vi "getparam.vi"(8 "error in (no error)":errorcluster, 11 "Input":string="34,45,89") -> (0 "error out":errorcluster, 3 "Output":string)   [LabVIEW 2014]
uses:
  <userlib>/Nanonis Prog Interface V5/Scan/Piezos/Piezo Calibration Range Get.vi
  <userlib>/Nanonis Prog Interface V5/Nanonis Prog Interface.lvlib
panel:
  out "size(s)":i32=3
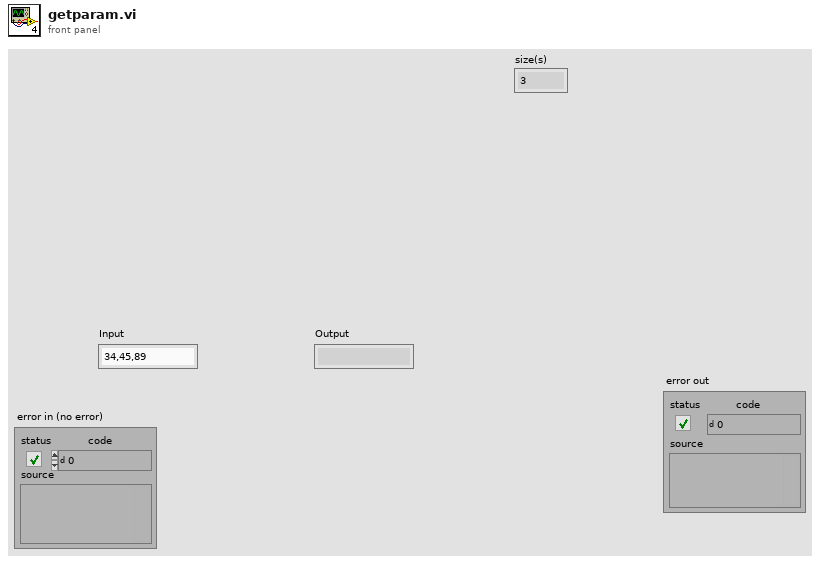
[diagram p1: front panel]
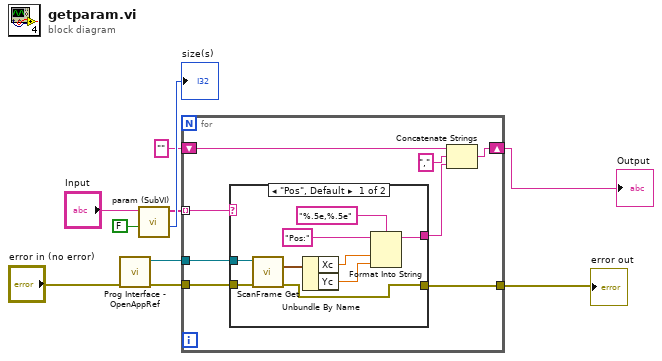
[diagram p0: block diagram]
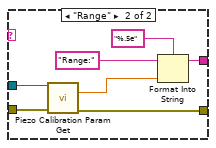
[diagram p2: hidden frame]
diagram:
  n1 = call <userlib>:"Prog Interface - OpenAppRef.vi"("Error in (no error)"="error in (no error)") -> ("Error out"=w3:errorcluster, "Application reference"=w5:refnum<vi>)  [unwired: 5 in]
  n2 = call <userlib>:"param (SubVI).vi"("Numeric"=FALSE, "Input"="Input") -> ("num"=→"size(s)":i32, "Array"=w6:string[])  [unwired: 7 in, 1 out]
  n3 = for {
    tunnel: w6 -> [w18] mode=indexing
    tunnel: w5 -> [w17]
    shift-right: [w13] -> w1
    shift-left: "" -> [w16]
    tunnel: w3 -> [w12]
    tunnel: [w11] -> w2
    n4 = case shown="\"Pos\", Default" w18 {
      tunnel: w17 -> [w27 w34]
      tunnel: [w20 w30] -> w14
      tunnel: w12 -> [w26 w29]
      tunnel: [w19 w28] -> w11
      frame "Pos", Default {
        n5 = call <userlib>:"ScanFrame Get.vi"("Application ref in"=w27, "error in (no error)"=w26) -> ("Center coordinates (m)"=w25:cluster{"Xc":sgl, "Yc":sgl}, "error out"=w19:errorcluster)  [unwired: 9 in, 3 out]
        n6 = Unbundle By Name(w25) -> ("Xc"=w22:sgl, "Yc"=w21:sgl)
        n7 = Format Into String(format string="%.5e,%.5e", initial string="Pos:", w22, w21) -> (resulting string=w20:string)  [unwired: 1 in, 1 out]
      }
      frame "Range" {
        n8 = call-poly <userlib>:"Piezo Calibration Param Get.vi"("Application ref in"=w34, "error in (no error)"=w29) -> ("Range X (m)"=w32:sgl, "error out"=w28:errorcluster)  [unwired: 9 in, 3 out]
        n9 = Format Into String(format string="%.5e", initial string="Range:", w32) -> (resulting string=w30:string)  [unwired: 1 in, 1 out]
      }
    }
    n10 = Concatenate Strings(w16, "," ("string"), w14) -> (w13:string)
  }
  "Output" <- w1
  "error out" <- w2
